vi "delete channel from TEC configuration.vi"(8 "error in":errorcluster, 10 "channel to delete":string, 11 "TEC configuration in":refnum<class "TEC configuration.lvclass">) -> (0 "error out":errorcluster, 3 "TEC configuration out":refnum<class "TEC configuration.lvclass">)   [LabVIEW 2013, in "TEC configuration.lvclass"]
uses:
  TEC configuration.lvclass
  TEC configuration.lvclass/TEC configuration.ctl
  <vilib>/NI/Tag Bus/tag/tag descriptor.lvclass/tag descriptor.ctl
  <vilib>/NI/Tag Bus/tag/read tag name.vi
  <vilib>/NI/Tag Bus/tag/tag descriptor.lvclass
  <vilib>/NI/Configuration Framework/NISE_CEF_TreeControl.lvlib
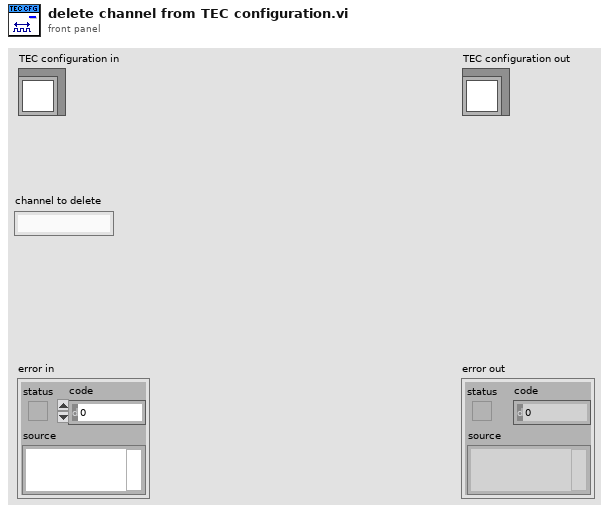
[diagram p1: front panel]
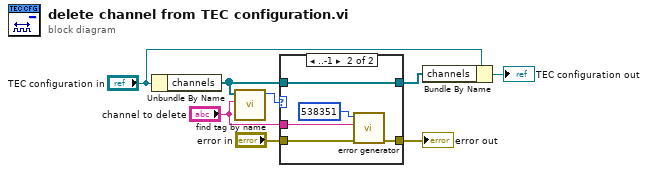
[diagram p0: block diagram]
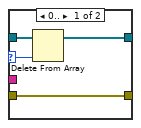
[diagram p2: hidden frame]
diagram:
  n1 = Unbundle By Name("TEC configuration in") -> ("channels"=w4:refnum<class "TBM channel.lvclass">[])
  n2 = call <vilib>:"find tag by name.vi"("name"="channel to delete", "tags in"=w4) -> ("index"=w6:i32)  [unwired: 9 in]
  n3 = case shown="..-1" w6 {
    selector: w6 -> [w11 _]
    tunnel: [w10 w16] -> w5
    tunnel: w4 -> [w12 w16]
    tunnel: "error in" -> [w9 w15]
    tunnel: [w9 w14] -> w2
    tunnel: "channel to delete" -> [_ w13]
    frame 0.. {
      n4 = Delete From Array(array=w12, index=w11) -> (array with subset deleted=w10:refnum<class "TBM channel.lvclass">[])  [unwired: 1 in, 1 out]
    }
    frame ..-1 {
      n5 = call <vilib>:"error generator.vi"("error in"=w15, "append error message"=w13, "error code (0)"=538351) -> ("error out"=w14:errorcluster)  [unwired: 6 in]
    }
  }
  "error out" <- w2
  n6 = Bundle By Name(cluster="TEC configuration in", "channels"=w5) -> (→"TEC configuration out":refnum<class "TEC configuration.lvclass">)
